vi "Read TS Front Panel Refnum.vi"(8 "error in (no error)":errorcluster, 11 "Display TS Panel in":refnum<class "UI Display TS Panel.lvclass">) -> (0 "error out":errorcluster, 2 "TS Front Panel Refnum":refnum<vi>, 3 "Display TS Panel out":refnum<class "UI Display TS Panel.lvclass">)   [LabVIEW 2019, in "User Interface Process.lvlib" / "UI Display TS Panel.lvclass"]
uses:
  UI Display TS Panel.lvclass
  UI Display TS Panel.lvclass/UI Display TS Panel.ctl
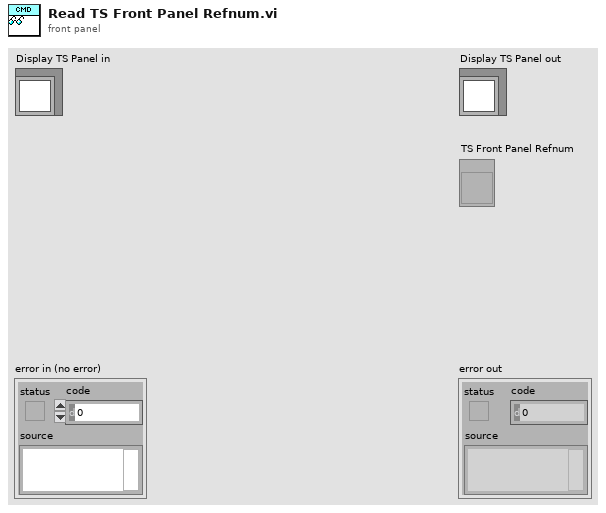
[diagram p1: front panel]
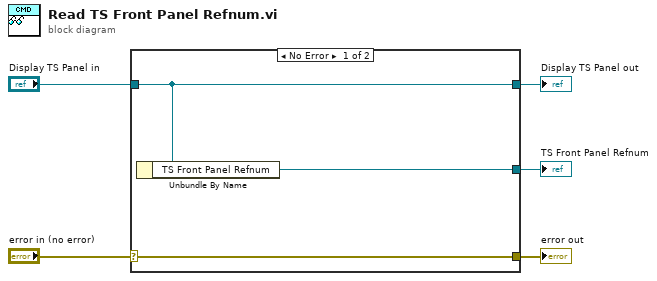
[diagram p0: block diagram]
diagram:
  n1 = case shown="No Error" "error in (no error)" {
    selector: "error in (no error)" -> [w8 w9]
    tunnel: [w8 w9] -> w4
    tunnel: [w7 w10] -> w2
    tunnel: "Display TS Panel in" -> [w7 w10]
    tunnel: [w6 _] -> w1
    frame No Error {
      n2 = Unbundle By Name(w7) -> ("TS Front Panel Refnum"=w6:refnum<vi>)
    }
    frame Error {
    }
  }
  "error out" <- w4
  "Display TS Panel out" <- w2
  "TS Front Panel Refnum" <- w1
